vi "Temperatura.vi"() -> ()   [LabVIEW 2015]
panel:
  out "Resultado 2":dbl
  out "Resultado":dbl
  in  "C":dbl
  in  "Bx":dbl
  in  "Ax^2":dbl
  out "Grados Kelvin":dbl
  in  "Grados Celcius":dbl
  out "C1":dbl
  in  "b":dbl
  in  "a":dbl
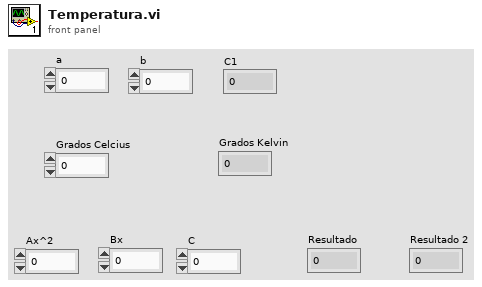
[diagram p1: front panel]
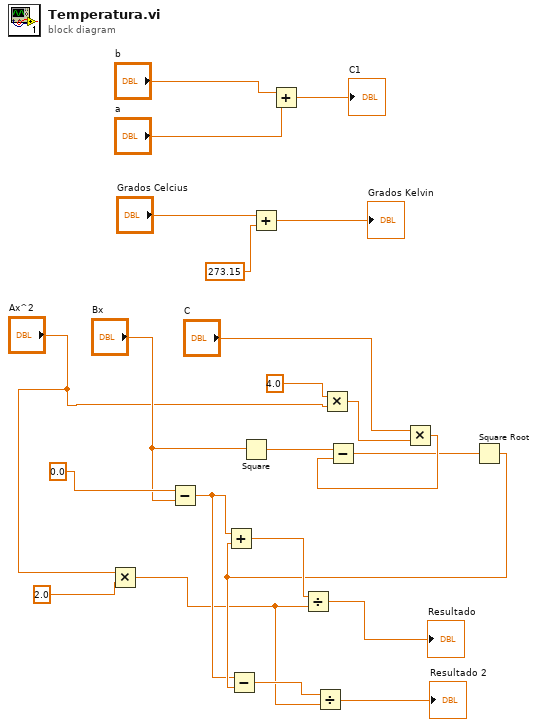
[diagram p0: block diagram]
diagram:
  n1 = Multiply(x="Ax^2", y=2.0) -> (x*y=w2:dbl)
  n2 = Subtract(x=0.0, y="Bx") -> (x-y=w3:dbl)
  n3 = Square(x="Bx") -> (x^2=w15:dbl)
  n4 = Add(x="Grados Celcius", y=273.15) -> (x+y=→"Grados Kelvin":dbl)
  n5 = Add(x="b", y="a") -> (x+y=→"C1":dbl)
  n6 = Multiply(x=4.0, y="Ax^2") -> (x*y=w12:dbl)
  n7 = Multiply(x="C", y=w12) -> (x*y=w11:dbl)
  n8 = Subtract(x=w15, y=w11) -> (x-y=w10:dbl)
  n9 = Square Root(x=w10) -> (sqrt(x)=w4:dbl)
  n10 = Add(x=w3, y=w4) -> (x+y=w9:dbl)
  n11 = Subtract(x=w3, y=w4) -> (x-y=w5:dbl)
  n12 = Divide(x=w9, y=w2) -> (x/y=→"Resultado":dbl)
  n13 = Divide(x=w5, y=w2) -> (x/y=→"Resultado 2":dbl)
